vi "Arduino input-output stand alone.vi"(4 "Sets to read":u32=1, 5 "VISA resource name":refnum<visa-resource-name>="COM18") -> (0 "Error out":errorcluster, 1 "Channel names":string[](array[string]), 2 "Output":dbl[][](array[numeric]))   [LabVIEW 2014]
uses:
  <vilib>/Instr/_visa.llb/VISA Configure Serial Port (Instr).vi
panel:
  out "Set Count":i32
  in  "stop":bool
  out "Time count":u32
  in  "Serial Settings":T1={"baud rate"=9600, "data bits"=8, "parity"=enum."None", "stop bits"=10, "flow control"=0, "Time out (ms)"=1000} {"flow control" items=["None"=0, "XON/XOFF"=1, "RTS/CTS"=2, "DTR/DSR"=4]; "stop bits" items=["1.0"=10, "1.5"=15, "2.0"=20]; "data bits" min=5 max=8 step=1; "baud rate" items=["75"=75, "110"=110, "134"=134, "150"=150, "300"=300, "600"=600, "1200"=1200, "1800"=1800, "2400"=2400, "4800"=4800, "7200"=7200, "9600"=9600, "14400"=14400, "19200"=19200, "28800"=28800, "38400"=38400, "56000"=56000, "57600"=57600, "115200"=115200, "128000"=128000, "230400"=230400]}
  in  "error in (no error)":errorcluster
  in  "Termination Character":u8=10 format="%.0x"
  out "String":string
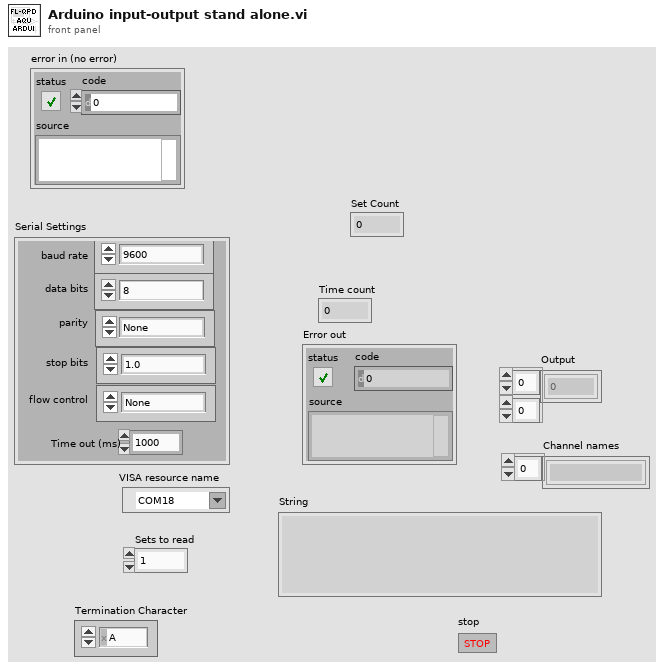
[diagram p1: front panel]
types:
  T1 = cluster{"baud rate":u32, "data bits":u16, "parity":enum16{"None", "Odd", "Even", "Mark", "Space"}, "stop bits":u16, "flow control":u16, "Time out (ms)":u32}
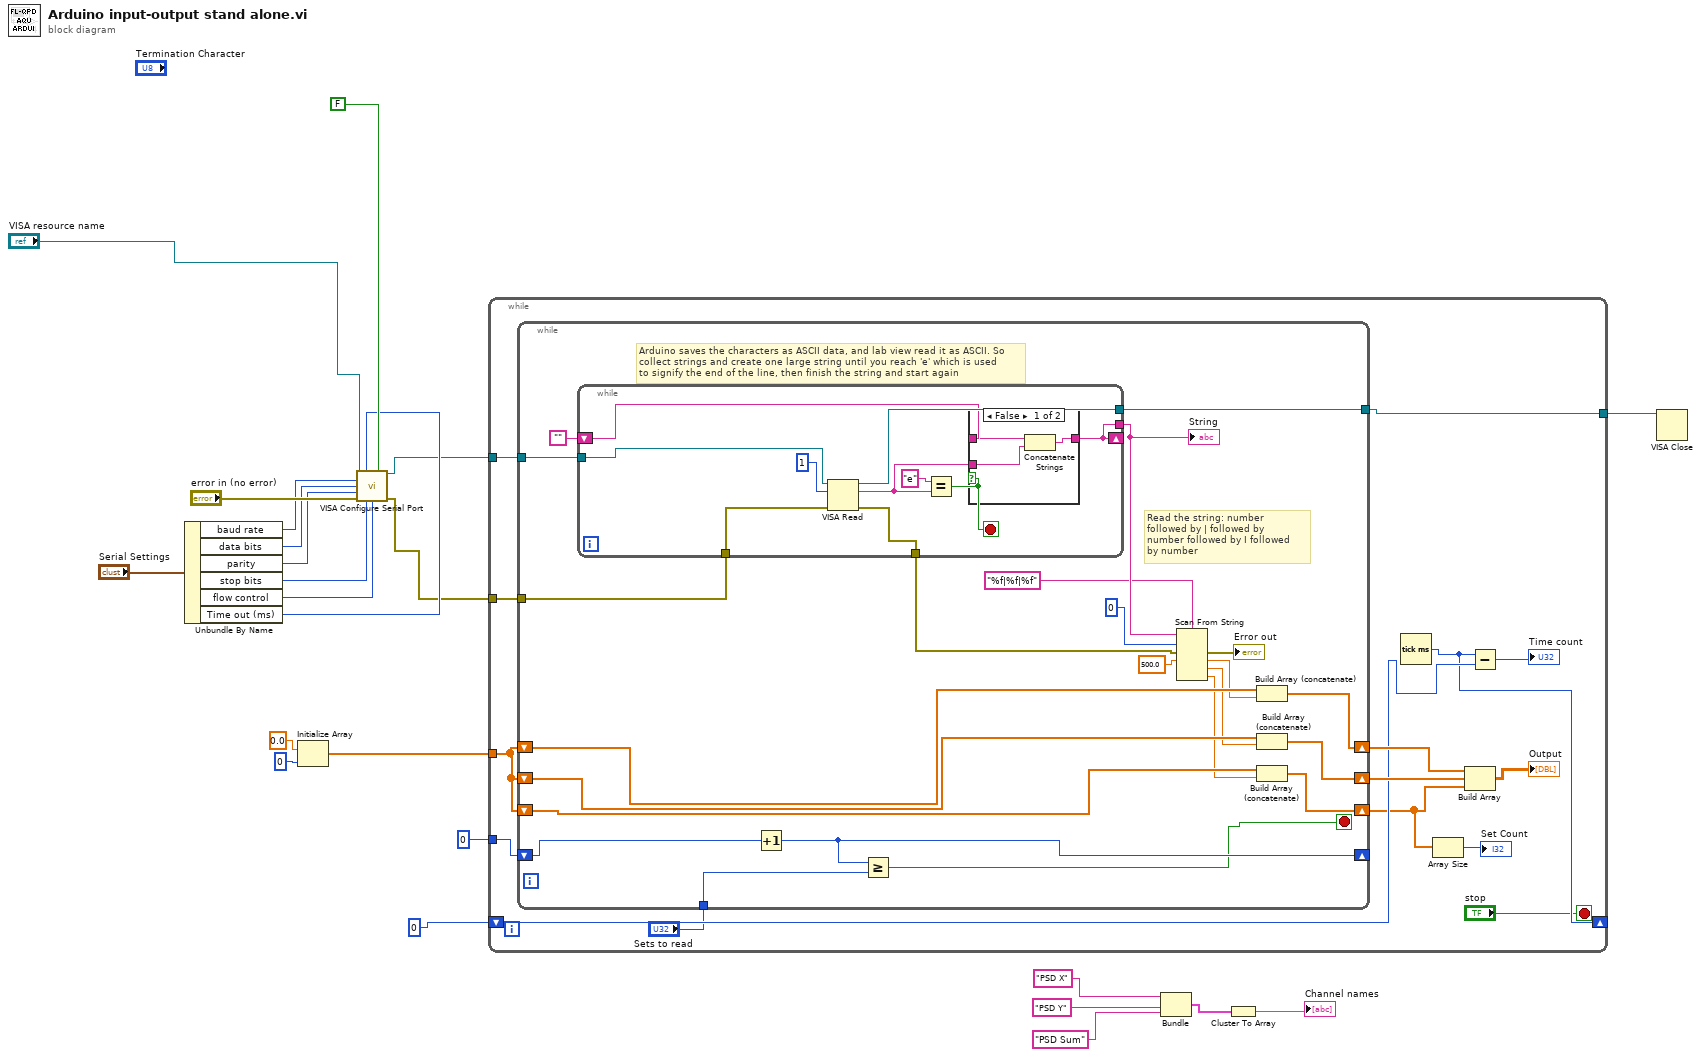
[diagram p0: block diagram]
diagram:
  n1 = Unbundle By Name("Serial Settings") -> ("baud rate"=w7:u32, "data bits"=w8:u16, "parity"=w9:enum16{"None", "Odd", "Even", "Mark", "Space"}, "stop bits"=w10:u16, "flow control"=w11:u16, "Time out (ms)"=w13:u32)
  n2 = Initialize Array(0.0, 0) -> (w20:dbl[])
  n3 = call-poly "VISA Configure Serial Port"("VISA resource name"="VISA resource name", "timeout (10sec)"=w13, "Enable Termination\nChar (T)"=FALSE, "baud rate (9600)"=w7, "data bits (8)"=w8, "parity (0:none)"=w9, "error in (no error)"="error in (no error)", "stop bits (10: 1 bit)"=w10, "flow control (0:none)"=w11) -> ("VISA resource name out"=w4:refnum<visa-resource-name>, "error out"=w3:errorcluster)  [unwired: 5 in]
  n4 = while {
    tunnel: u32 0 -> [w38]
    tunnel: w20 -> [w37]
    tunnel: w4 -> [w33]
    tunnel: w3 -> [w32]
    tunnel: [w31] -> w2
    shift-right: [w28] -> _
    shift-left: u32 0 -> [w29]
    stop <- "stop" stop-if-true
    n5 = while {
      tunnel: w33 -> [w53]
      tunnel: [w61] -> w31
      tunnel: w32 -> [w54]
      shift-right: [w51] -> _
      shift-left: w38 -> [w52]
      tunnel: "Sets to read" -> [w50]
      shift-right: [w43] -> w36
      shift-left: w37 -> [w49]
      shift-right: [w42] -> w35
      shift-left: w37 -> [w47]
      shift-right: [w41] -> w25
      shift-left: w37 -> [w45]
      stop <- w39 stop-if-true
      # "Read the string: number \nfollowed by | followed by\nnumber followed by I followed \nby number"
      # "Arduino saves the characters as ASCII data, and lab view read it as ASCII. So\ncollect strings and create one large string until you reach 'e' which is used \nto signify the end of the line, then finish the string and start again"
      n6 = while {
        tunnel: [w64] -> w59
        tunnel: w53 -> [w71]
        tunnel: [w69] -> w61
        shift-right: [w64] -> _
        shift-left: "" -> [w65]
        tunnel: w54 -> [w63]
        tunnel: [w62] -> w40
        stop <- w66 stop-if-true
        n7 = VISA Read(VISA resource name=w71, byte count=1, error in (no error)=w63) -> (VISA resource name out=w69:refnum<visa-resource-name>, read buffer=w67:string, error out=w62:errorcluster)  [unwired: 1 out]
        n8 = Equal?(x="e", y=w67) -> (x = y?=w66:bool)
        n9 = case shown="False" w66 {
          tunnel: w65 -> [w74 w75]
          tunnel: w67 -> [w73 _]
          tunnel: [w72 w75] -> w64
          frame False {
            n10 = Concatenate Strings(w74, w73) -> (w72:string)
          }
          frame True {
          }
        }
      }
      "String" <- w59
      n11 = Increment(x=w52) -> (x+1=w51:u32)
      n12 = Greater Or Equal?(x=w51, y=w50) -> (x >= y?=w39:bool)
      n13 = Scan From String(format string="%f|%f|%f", input string=w59, initial scan location=0, error in=w40, default 1=500.0) -> (error out=→"Error out":errorcluster, output 1=w48:dbl, output 2=w46:dbl, output 3=w44:dbl)  [unwired: 2 in, 2 out]
      n14 = Build Array (concatenate)(w49, w48) -> (w43:dbl[])
      n15 = Build Array (concatenate)(w47, w46) -> (w42:dbl[])
      n16 = Build Array (concatenate)(w45, w44) -> (w41:dbl[])
    }
    n17 = Tick Count (ms)() -> (millisecond timer value=w28:u32)
    n18 = Array Size(array=w25) -> (size(s)=→"Set Count":i32)
    n19 = Build Array(w36, w35, w25) -> (→"Output":dbl[][])
    n20 = Subtract(x=w28, y=w29) -> (x-y=→"Time count":u32)
  }
  n21 = Bundle("PSD X", "PSD Y", "PSD Sum") -> (w16:cluster{string, string, string})  [unwired: 1 out]
  n22 = Cluster To Array(cluster=w16) -> (array=→"Channel names":string[])
  n23 = VISA Close(VISA resource name=w2) -> ()  [unwired: 1 in, 1 out]
